vi "clear picture.vi"(7 "Keep Keyboard? (T)":bool=TRUE, 8 "error in":errorcluster, 11 "midi-ui in":refnum<class "midi-ui.lvclass">) -> (0 "error out":errorcluster, 3 "midi-ui out":refnum<class "midi-ui.lvclass">)   [LabVIEW 2020, in "midi-ui.lvclass"]
uses:
  midi-ui.lvclass
  midi-ui.lvclass/midi-ui.ctl
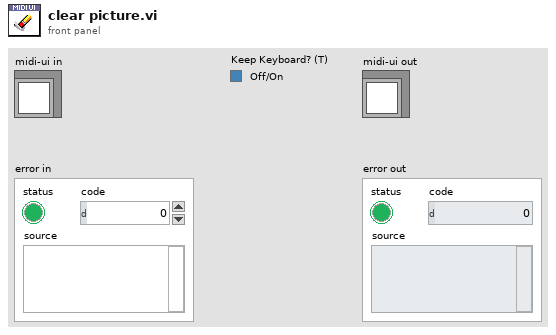
[diagram p1: front panel]
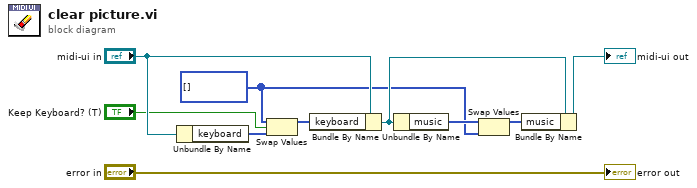
[diagram p0: block diagram]
diagram:
  w1 = picture[] []
  n1 = Unbundle By Name("midi-ui in") -> ("keyboard"=w7:picture[])
  n2 = Swap Values(12:w1, 13:"Keep Keyboard? (T)", 14:w7) -> (1:w9:picture[])  [unwired: 1 out]
  n3 = Bundle By Name(cluster="midi-ui in", "keyboard"=w9) -> (w4:refnum<class "midi-ui.lvclass">)
  n4 = Unbundle By Name(w4) -> ("music"=w5:picture[])
  n5 = Swap Values(12:w5, 14:w1) -> (1:w6:picture[])  [unwired: 1 in, 1 out]
  n6 = Bundle By Name(cluster=w4, "music"=w6) -> (→"midi-ui out":refnum<class "midi-ui.lvclass">)
  "error out" <- "error in"
